vi "Write to Coil Channels.vi"(8 "error in (no error)":errorcluster, 9 "Coils":T1[](array[typedef]), 10 "Data In":dbl[](array[numeric]), 11 "Modbus Master in":refnum<class "Modbus Master.lvclass">) -> (0 "error out":errorcluster, 2 "Data Out":dbl[](array[numeric]), 3 "Modbus Master out":refnum<class "Modbus Master.lvclass">)   [LabVIEW 2015]
uses:
  Modbus API.lvlibp/API/Master/Modbus Master.lvclass
  Shared/Controls/Data Model/Channel.ctl
  System Explorer/SubVIs/Modbus Type.ctl
  <vilib>/NI Veristand/Custom Device API/Custom Device Channel Type.ctl
  Shared/Controls/Data Model/Mapping.ctl
  Shared/Controls/Data Model/DataType.ctl
  <vilib>/NI Veristand/Custom Device API/Custom Device Item Ref.ctl
  Shared/Modbus Master Shared.lvlib
  <vilib>/NI VeriStand/Custom Device API/Custom Device API.lvlib
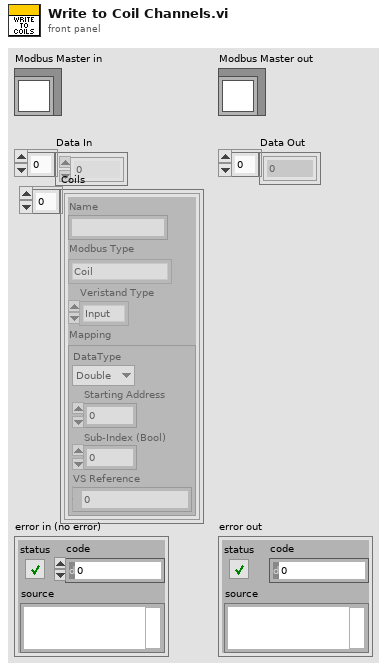
[diagram p1: front panel]
types:
  T1 = typedef "Modbus Master Shared.lvlib/Channel.ctl" = cluster{"Name":string, "Modbus Type":T2, "Veristand Type":T3, "Mapping":T4}
  T2 = typedef "Modbus Master Shared.lvlib/Modbus Type.ctl" = enum16{"Coil", "Discrete Input", "Holding Register", "Input Register"}
  T3 = typedef "Custom Device API.lvlib/Custom Device Channel Type.ctl" = enum16{"Input", "Output"}
  T4 = typedef "Modbus Master Shared.lvlib/Mapping.ctl" = cluster{"DataType":T5, "Starting Address":u16, "Sub-Index (Bool)":u16, "VS Reference":T6}
  T5 = typedef "Modbus Master Shared.lvlib/DataType.ctl" = enum16{"Double", "Single", "I64", "I32", "I16", "I8", "U64", "U32", "U16", "U8", "Boolean"}
  T6 = typedef "Custom Device API.lvlib/Custom Device Item Ref.ctl" = u64
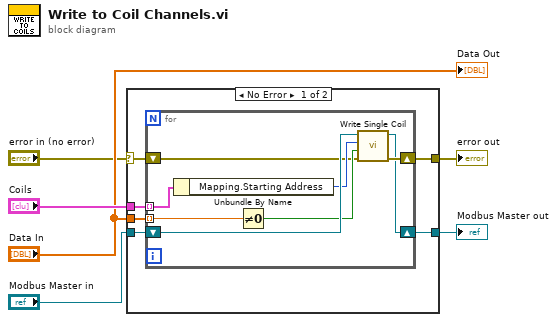
[diagram p0: block diagram]
diagram:
  n1 = case shown="No Error" "error in (no error)" {
    selector: "error in (no error)" -> [w8 w22]
    tunnel: [w12 w22] -> w6
    tunnel: [w11 w21] -> w5
    tunnel: "Coils" -> [w10 _]
    tunnel: "Data In" -> [w9 _]
    tunnel: "Modbus Master in" -> [w7 w21]
    frame No Error {
      n2 = for {
        tunnel: w10 -> [w19] mode=indexing
        tunnel: w9 -> [w17] mode=indexing
        shift-right: [w13] -> w11
        shift-left: w7 -> [w20]
        shift-right: [w14] -> w12
        shift-left: w8 -> [w15]
        n3 = Unbundle By Name(w19) -> ("Mapping.Starting Address"=w18:u16)
        n4 = Not Equal To 0?(x=w17) -> (x != 0?=w16:bool)
        n5 = call-dynamic "Write Single Coil.vi"("error in"=w15, "coil to write"=w16, "address"=w18, "Modbus master in"=w20) -> ("error out"=w14:errorcluster, "Modbus master out"=w13:refnum<class "Modbus Master.lvclass">)  [unwired: 6 in]
      }
    }
    frame Error {
    }
  }
  "error out" <- w6
  "Modbus Master out" <- w5
  "Data Out" <- "Data In"
